vi "All Groups.vi"(8 "error in (no error)":errorcluster, 11 "ChannelService in":refnum<class "ChannelService.lvclass">) -> (0 "error out":errorcluster, 2 "Groups":refnum<class "Group.lvclass">[](array[class]), 3 "ChannelService out":refnum<class "ChannelService.lvclass">)   [LabVIEW 2020, in "Vecto.lvlib" / "ChannelService.lvclass"]
uses:
  ChannelService.lvclass
  Group/Group.lvclass
  GroupsAbstractValue/GroupsAbstractValue.lvclass
  C:/dev/lv20CE/relink/lv-promises/Promises/Value/Value.lvclass
  ChannelService.lvclass/ChannelService.ctl
  lv-promises/Promises/Promise/Promise.lvclass/Promise.ctl
  lv-promises/Promises/Future/Future.lvclass/Future.ctl
  GroupsAbstractValue/GroupsAbstractValue.lvclass/GroupsAbstractValue.ctl
  lv-promises/Promises/Future/Future.lvclass
  lv-promises/Promises/Promise/Promise.lvclass
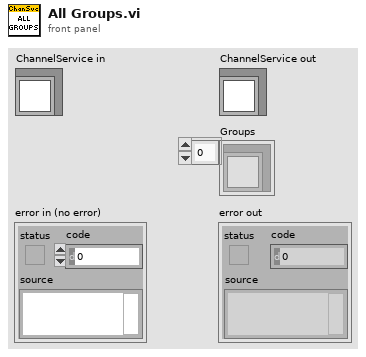
[diagram p1: front panel]
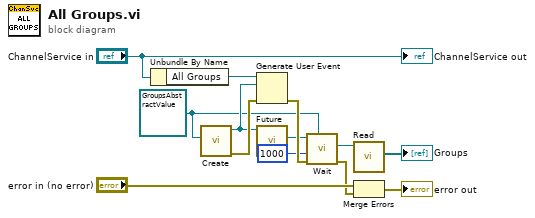
[diagram p0: block diagram]
diagram:
  w6 = refnum<class "GroupsAbstractValue.lvclass"> refnum ("Vecto.lvlib:GroupsValue.lvclass")
  n1 = Unbundle By Name("ChannelService in") -> ("All Groups"=w9:refnum<user-event>)
  n2 = call "Create.vi"("Result Type"=w6) -> ("error out"=w12:errorcluster, "Promise"=w8:refnum<class "Promise.lvclass">)  [unwired: 9 in]
  n3 = Generate User Event(user event=w9, event data cluster=w8, error in=w12) -> (error out=w13:errorcluster)  [unwired: 1 in, 1 out]
  n4 = call "Future.vi"("Promise in"=w8) -> ("Future"=w7:refnum<class "Future.lvclass">)  [unwired: 9 in, 1 out]
  n5 = call "Wait.vi"("Result Type"=w6, "error in (no error)"=w13, "Timeout mS (-1)"=1000, "Future in"=w7) -> ("error out"=w1:errorcluster, "Result"=w4:refnum<class "GroupsAbstractValue.lvclass">)  [unwired: 6 in]
  n6 = call "Read.vi"("GroupsAbstractValue in"=w4) -> ("Groups"=→"Groups":refnum<class "Group.lvclass">[])  [unwired: 10 in]
  n7 = Merge Errors("error in (no error)", w1) -> (→"error out":errorcluster)
  "ChannelService out" <- "ChannelService in"
